vi "Heartbeat start.vi"(4 "error in":errorcluster, 6 "Node ID":u8, 7 "CANopen in":refnum<class "CANopen.lvclass">) -> (0 "error out":errorcluster, 3 "CANopen out":refnum<class "CANopen.lvclass">)   [LabVIEW 2024, in "canopen.lvlib" / "CANopen.lvclass"]
doc: "Starts the generation of heartbeat messages from a specific node or from all the nodes stored in the heartbeat table if \"Node ID\" is not specified."
uses:
  CANopen.lvclass
  CANopen.lvclass/CANopen.ctl
  Multiplexor.ctl
  SDO download (U16).vi
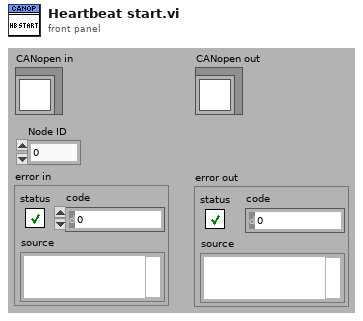
[diagram p1: front panel]
types:
  T1 = cluster{"Node ID":u8, "Period":dbl, "Set value":i16, "Value":i16}[]
  T2 = typedef "canopen.lvlib/CANopen.lvclass/Multiplexor.ctl" = cluster{"Index":u16, "Sub-index":u8}
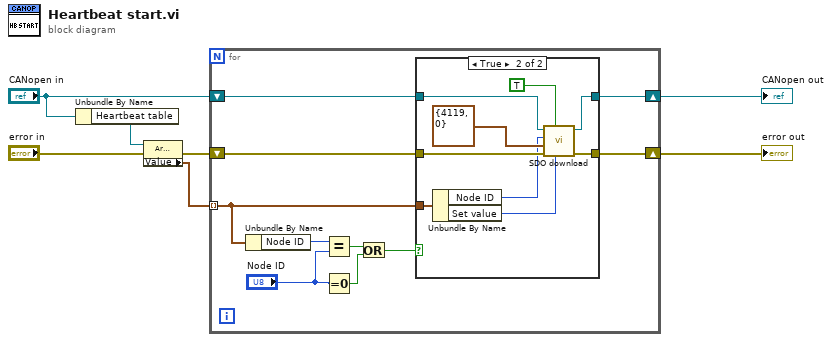
[diagram p0: block diagram]
diagram:
  n1 = Unbundle By Name("CANopen in") -> ("Heartbeat table"=w7:refnum<vi>)
  n2 = property class="Arr (strict)"(reference=w7, error in="error in") -> (error out=w3:errorcluster, "Value"=w6:T1)  [unwired: 1 out]
  n3 = for {
    tunnel: w6 -> [w10] mode=indexing
    shift-right: [w13] -> w2
    shift-left: w3 -> [w14]
    shift-right: [w8] -> w1
    shift-left: "CANopen in" -> [w12]
    n4 = Unbundle By Name(w10) -> ("Node ID"=w11:u8)
    n5 = Equal?(x=w11, y="Node ID") -> (x = y?=w16:bool)
    n6 = Equal To 0?(x="Node ID") -> (x = 0?=w15:bool)
    n7 = Or(x=w16, y=w15) -> (x .or. y?=w9:bool)
    n8 = case shown="True" w9 {
      tunnel: w14 -> [w19 w28]
      tunnel: [w19 w27] -> w13
      tunnel: w12 -> [w18 w23]
      tunnel: w10 -> [_ w25]
      tunnel: [w18 w22] -> w8
      frame False {
      }
      frame True {
        n9 = Unbundle By Name(w25) -> ("Node ID"=w21:u8, "Set value"=w24:i16)
        n10 = call-poly "SDO download.vi"("Value"=w24, "Wait?"=TRUE, "error in (no error)"=w28, "Multiplexor"=T2 {"Index"=4119, "Sub-index"=0}, "Node ID"=w21, "CANopen in"=w23) -> ("error out"=w27:errorcluster, "CANopen out"=w22:refnum<class "CANopen.lvclass">)  [unwired: 2 out]
      }
    }
  }
  "CANopen out" <- w1
  "error out" <- w2
